vi "construct G code string.vi"(6 "Speed":i32, 7 "ZF":dbl, 8 "YF":dbl, 9 "XF":dbl) -> (3 "GCode":string)   [LabVIEW 2014, in "HPCNC.lvlib"]
uses:
  HPCNC.lvlib
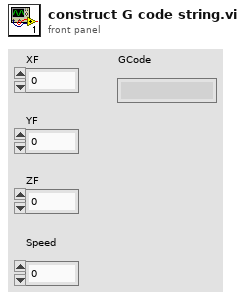
[diagram p1: front panel]
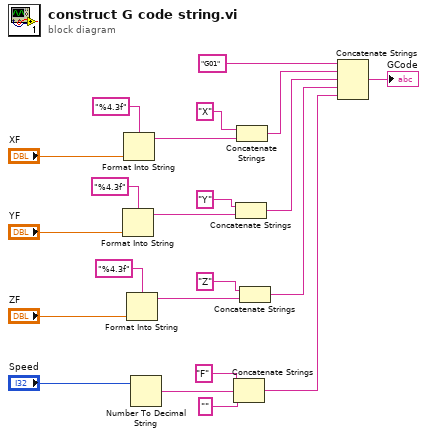
[diagram p0: block diagram]
diagram:
  n1 = Format Into String(format string="%4.3f", "YF") -> (resulting string=w12:string)  [unwired: 2 in, 1 out]
  n2 = Format Into String(format string="%4.3f", "XF") -> (resulting string=w17:string)  [unwired: 2 in, 1 out]
  n3 = Format Into String(format string="%4.3f", "ZF") -> (resulting string=w7:string)  [unwired: 2 in, 1 out]
  n4 = Number To Decimal String(number="Speed") -> (decimal integer string=w2:string)  [unwired: 1 in]
  n5 = Concatenate Strings("F" ("string"), w2, "" ("string")) -> (w1:string)
  n6 = Concatenate Strings("Y" ("string"), w12) -> (w11:string)
  n7 = Concatenate Strings("X" ("string"), w17) -> (w16:string)
  n8 = Concatenate Strings("Z" ("string"), w7) -> (w6:string)
  n9 = Concatenate Strings("G01" ("string"), w16, w11, w6, w1) -> (→"GCode":string)
